vi "P3 Side.vi"(0 "Image In":T1, 1 "File Path (Grid Calibration)":path=path "C:/Users/serce/Desktop/Smart Vision System Testbench/Grid Calibration.png", 2 "Template File Path (Locate P3 Hole)":path=path "C:/Users/serce/Desktop/Smart Vision System Testbench/P3 Side/P3 Side Template.png", 7 "error in":errorcluster) -> (20 "Image Out":T1, 21 "Number of Matches (Locate P3 Hole)":i32, 22 "Fitted Circle (P3 Hole)":T2 {"Average SNR (dB)" format="%.2f"; "Average Strength" format="%.2f"; "Roundness (Real-World)" format="%.2f"; "Radius (Real-World)" format="%.2f"; "Center (Real-World)"."Y" format="%.2f"; "Center (Real-World)"."X" format="%.2f"; "Radius (Pixels)" format="%.2f"; "Center (Pixels)"."Y" format="%.2f"; "Center (Pixels)"."X" format="%.2f"}, 23 "Calibrated Results (P3 Side Top Length)":sgl[][](array[numeric]) format="%.2f", 27 "error out":errorcluster)   [LabVIEW 2020]
uses:
  <vilib>/vision/Image Controls.llb/IMAQ Image.ctl
  <vilib>/vision/Pattern Matching.llb/IMAQ Curve Parameters.ctl
  <vilib>/vision/Pattern Matching.llb/IMAQ Match Range Setting.ctl
  <vilib>/vision/Pattern Matching.llb/IMAQ Geometric Pattern 2 Advanced Match Options.ctl
  <vilib>/vision/Image Controls.llb/Vision Info Type2.ctl
  <vilib>/vision/Measure.llb/Edge Options.ctl
  <vilib>/vision/Measure.llb/Edge Polarity.ctl
  <vilib>/vision/NI_Vision_Development_Module.lvlib
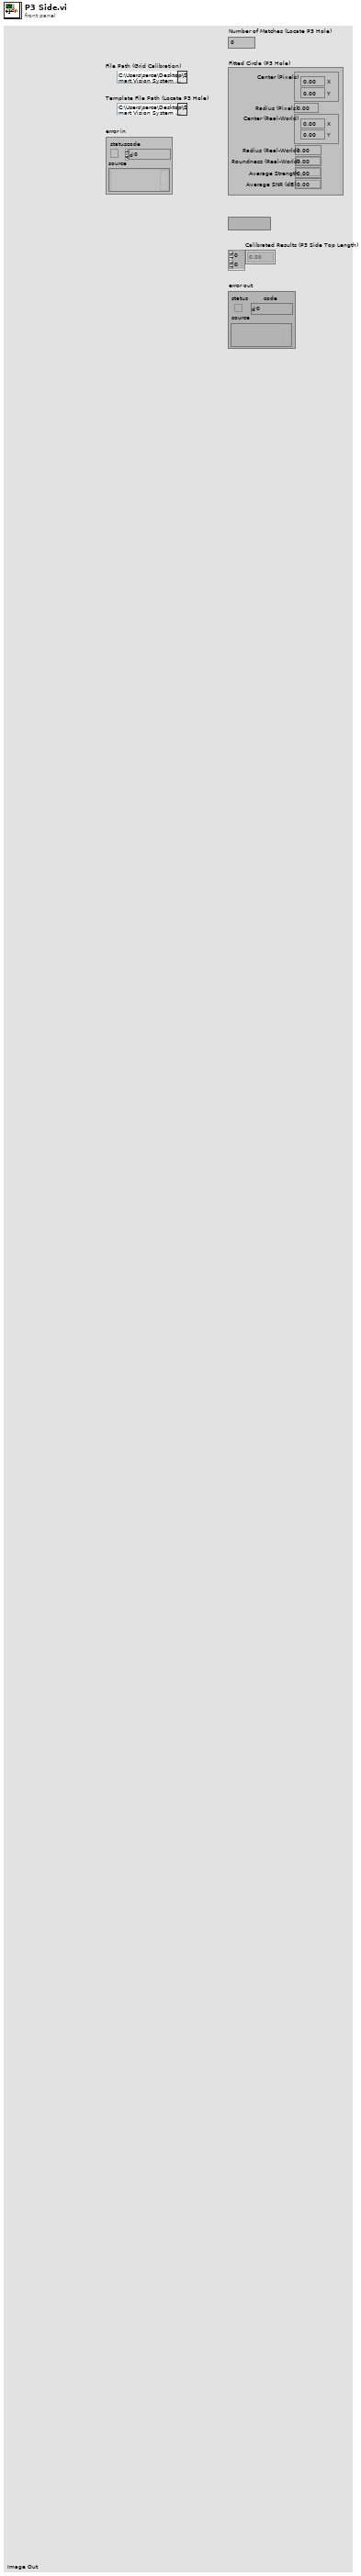
[diagram p1: front panel]
types:
  T1 = typedef "IMAQ Image.ctl" = refnum<image>
  T2 = cluster{"Center (Pixels)":cluster{"X":sgl, "Y":sgl}, "Radius (Pixels)":dbl, "Center (Real-World)":cluster{"X":sgl, "Y":sgl}, "Radius (Real-World)":dbl, "Roundness (Real-World)":dbl, "Average Strength":dbl, "Average SNR (dB)":dbl}
  T3 = cluster{"Feature":u32, "Points IDs":cluster{"GUID":string, "Index":i32}[]}[]
  T4 = cluster{"Edge Polarity":u32, "Kernel Size":u32, "Width":u32, "Minimum Edge Strength":sgl, "Interpolation Type":enum32{"Zero Order", "Bilinear", "Quadratic", "Cubic", "Bilinear Fixed"}, "Data Processing Method":enum32{"Average", "Median"}}
  T5 = enum16{"Get First Edge", "Get First + Last Edge", "Get All Edges", "Get Best Edge"}
  T6 = cluster{"Global Rectangle":i32[], "Contours":cluster{"ID":enum32{"External", "Internal"}, "Type":u32, "Coordinates":i32[]}[]}
  T7 = cluster{"Origin":cluster{"X":sgl, "Y":sgl}, "Angle (deg)":sgl, "Axis Reference":u32}
  T8 = enum16{"Reset", "Update Coordinate System", "Get Coordinate System"}
  T9 = typedef "Edge Options.ctl" = cluster{"Edge Polarity":T10, "Kernel Size":u32, "Width":u32, "Minimum Edge Strength":sgl, "Interpolation Type":enum32{"Zero Order", "Bilinear", "Quadratic", "Cubic", "Bilinear Fixed"}, "Data Processing Method":enum32{"Average", "Median"}}
  T10 = typedef "Edge Polarity.ctl" = u32
  T11 = cluster{"Search  Direction":u32, "Edge Options":T9, "Show Search Area":bool, "Show Search Lines":bool, "Show Edges Found":bool, "Show Result":bool, "Search Area Color":u32, "Search Lines Color":u32, "Edge Locations Color":u32, "Result Color":u32, "Overlay Group Name":string}
  T12 = cluster{"Process":enum16{"Get First Edge", "Get First + Last Edge", "Get All Edges", "Get Best Edge"}, "Step Size":i32, "Max Pixel Radius":i32}
  T13 = cluster{"Origin Pixel":cluster{"X":sgl, "Y":sgl}, "X Axis Pixel":cluster{"X":sgl, "Y":sgl}, "Axis Reference":u32}
  T14 = typedef "Vision Info Type2.ctl" = u32
  T15 = typedef "Simple Grid Descriptor" = cluster{"X Step":sgl, "Y Step":sgl, "Unit":T16}
  T16 = typedef "Image Unit" = enum32{"Undefined", "Angström", "Micrometer", "Millimeter", "Centimeter", "Meter", "Kilometer", "Microinch", "Inch", "Feet", "Nautical miles", "Standard miles", "Steps"}
  T17 = enum16{"Horizontal Motion", "Vertical Motion", "Horizontal and Vertical Motion", "Horizontal, Vertical and Angular Motion"}
  T18 = typedef "IMAQ Curve Parameters.ctl" = cluster{"Extraction Mode":u32, "Edge Threshold":i32, "Edge Filter Size":u32, "Min Length":i32, "Row Search Step Size":i32, "Col Search Step Size":i32, "Max Endpoint Gap":i32, "Closed":bool, "Subpixel":bool}
  T19 = typedef "IMAQ Match Range Setting.ctl" = cluster{"Match Constraints":u32, "Min":dbl, "Max":dbl}
  T20 = typedef "IMAQ Geometric Pattern 2 Advanced Match Options.ctl" = u16
  T21 = cluster{"Curve Parameters":T18, "Match Mode":cluster{"Rotation":bool, "Scale":bool, "Occlusion":bool, "Reserved 1":bool, "Reserved 2":bool, "Reserved 3":bool}, "Range Settings":T19[], "Number of Matches":i32, "Minimum Match Score":sgl, "SubPixel Accuracy":bool, "Adv. Geometric Match Options 2":cluster{"Setup Data Item":T20, "Item Value":dbl}[]}
  T22 = cluster{"Brightness":sgl, "Contrast":sgl, "Gamma":sgl}
  T23 = typedef "IMAQ GM Match Report.ctl" = cluster{"Position":cluster{"x":sgl, "y":sgl}, "Angle":sgl, "Scale":sgl, "Score":sgl, "Bounding Box":cluster{"x":sgl, "y":sgl}[], "Contrast Reversed":bool, "Occlusion %":sgl, "Template Target Curve Score":sgl, "Target Template Curve Score":sgl, "Correlation Score":sgl}
  T24 = typedef "IMAQ Coordinate System" = cluster{"Reference System":cluster{"Origin":cluster{"X":sgl, "Y":sgl}, "Angle (deg)":sgl, "Axis Reference":u32}, "Measurement System":cluster{"Origin":cluster{"X":sgl, "Y":sgl}, "Angle (deg)":sgl, "Axis Reference":u32}}
  T25 = typedef "ROI Descriptor" = cluster{"Global Rectangle":i32[], "Contours":cluster{"ID":enum32{"External", "Internal"}, "Type":u32, "Coordinates":i32[]}[]}
  T26 = typedef "Edge New.ctl" = cluster{"Location (Pixel)":cluster{"X":sgl, "Y":sgl}, "Location (Real-World)":cluster{"X":sgl, "Y":sgl}, "Distance (Pixel)":dbl, "Distance (Real-World)":dbl, "Strength":dbl, "Noise":dbl, "Rising?":bool}
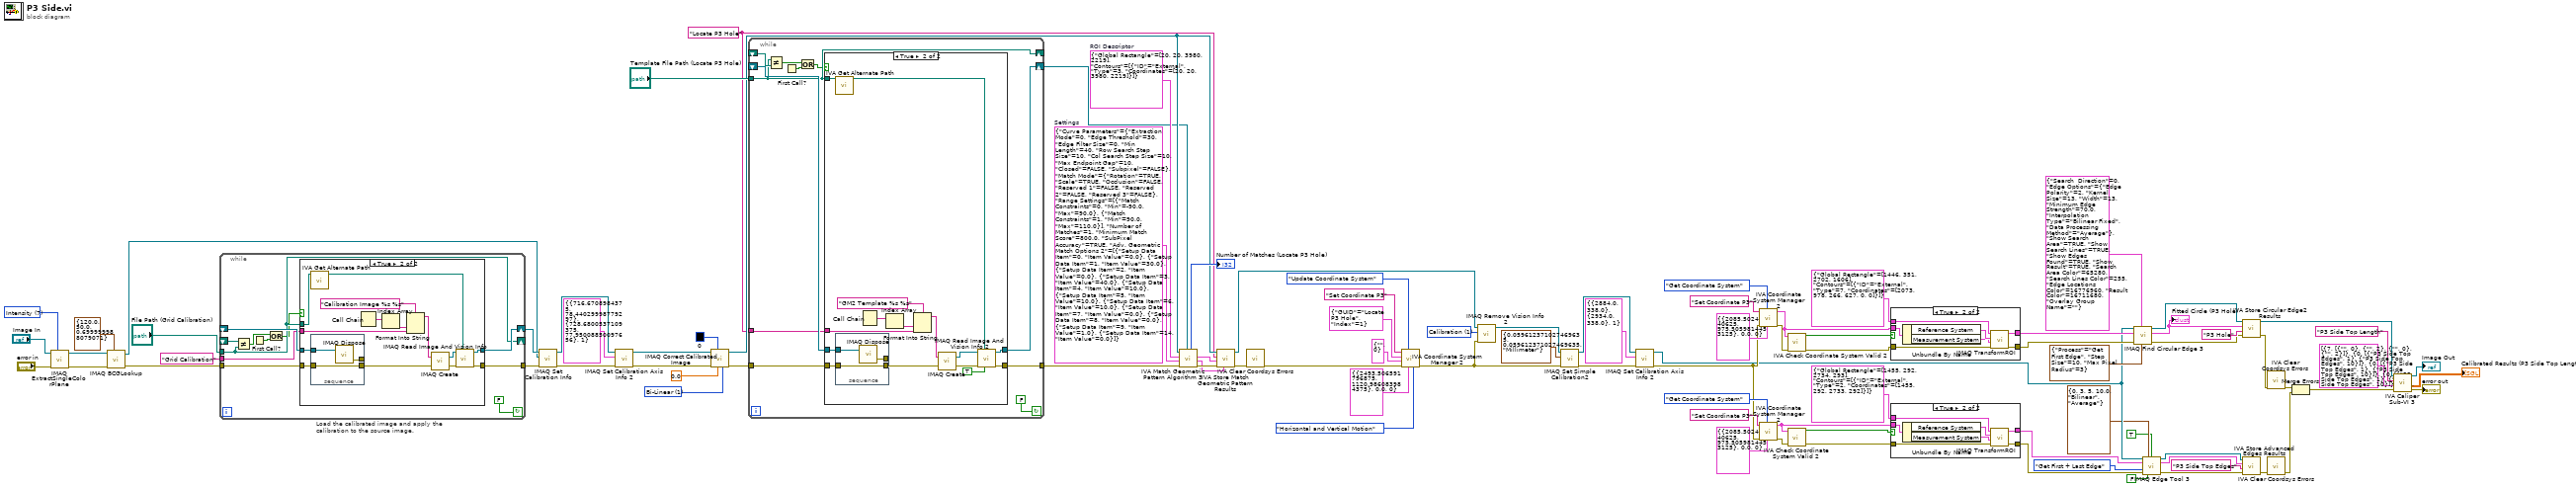
[diagram p0: block diagram]
diagram:
  w54 = T14 1 items=["Any", "Calibration", "Overlay", "Grayscale Template", "Color Template", "Geometric Template", "Custom Data", "Golden Template", "Geometric Template 2", "Contour Data", "Camera Model"] ("Vision Info")
  w67 = T21 {"Curve Parameters"={"Extraction Mode"=0, "Edge Threshold"=30, "Edge Filter Size"=0, "Min Length"=40, "Row Search Step Size"=10, "Col Search Step Size"=10, "Max Endpoint Gap"=10, "Closed"=FALSE, "Subpixel"=FALSE}, "Match Mode"={"Rotation"=TRUE, "Scale"=TRUE, "Occlusion"=FALSE, "Reserved 1"=FALSE, "Reserved 2"=FALSE, "Reserved 3"=FALSE}, "Range Settings"=[{"Match Constraints"=0, "Min"=-90.0, "Max"=90.0}, {"Match Constraints"=1, "Min"=90.0, "Max"=110.0}], "Number of Matches"=1, "Minimum Match Score"=800.0, "SubPixel Accuracy"=TRUE, "Adv. Geometric Match Options 2"=[{"Setup Data Item"=0, "Item Value"=0.0}, {"Setup Data Item"=1, "Item Value"=30.0}, {"Setup Data Item"=2, "Item Value"=0.0}, {"Setup Data Item"=3, "Item Value"=40.0}, {"Setup Data Item"=4, "Item Value"=10.0}, {"Setup Data Item"=5, "Item Value"=10.0}, {"Setup Data Item"=6, "Item Value"=10.0}, {"Setup Data Item"=7, "Item Value"=0.0}, {"Setup Data Item"=8, "Item Value"=0.0}, {"Setup Data Item"=9, "Item Value"=1.0}, {"Setup Data Item"=14, "Item Value"=0.0}]}  # Settings
  w66 = "Locate P3 Hole" ("Step Name")
  w74 = T6 {"Global Rectangle"=[20, 20, 3980, 2219], "Contours"=[{"ID"=enum."External", "Type"=3, "Coordinates"=[20, 20, 3980, 2219]}]}  # ROI Descriptor
  w80 = u32 1 items=["Zero Order", "Bi-Linear", "Quadratic", "Cubic Spline"] ("Interpolation Type")
  w95 = 7 items=["Red", "Green", "Blue", "Hue", "Saturation", "Luminance", "Value", "Intensity"] ("Color Plane")
  n1 = call "IMAQ ExtractSingleColorPlane"("Color Plane"=w95, "error in (no error)"="error in", "Image Src"="Image In") -> ("error out"=w91:errorcluster, "Image Dst Out"=w92:T1)  [unwired: 1 in, 6 out]
  n2 = call "IMAQ BCGLookup"("Image Src"=w92, "BCG Values"=T22 {"Brightness"=120.0, "Contrast"=50.0, "Gamma"=0.7}, "error in (no error)"=w91) -> ("Image Dst Out"=w85:T1, "error out"=w89:errorcluster)  [unwired: 2 in, 2 out]
  n3 = while "Load the calibrated image and apply the calibration to the source image." {
    shift-right: [w106] -> w87
    shift-left: _ -> [w105]
    tunnel: [w103] -> w86
    tunnel: w89 -> [w102]
    tunnel: "File Path (Grid Calibration)" -> [w99]
    tunnel: "Grid Calibration" ("Step Name") -> [w101]
    shift-right: [w99] -> _
    shift-left: _ -> [w100]
    stop <- FALSE continue-if-true
    n4 = Not Equal?(x=w100, y=w99) -> (x != y?=w97:bool)
    n5 = First Call?() -> (First Call?: T/F=w98:bool)
    n6 = Or(x=w97, y=w98) -> (x .or. y?=w96:bool)
    n7 = case shown="True" w96 {
      tunnel: [w108 w120] -> w106
      tunnel: w105 -> [w108 w112]
      tunnel: [w107 w117] -> w103
      tunnel: w102 -> [w107 w113]
      tunnel: w99 -> [_ w110]
      tunnel: w101 -> [_ w114]
      frame False {
      }
      frame True {
        n8 = call <vilib>:"IVA Get Alternate Path.vi"("Path In"=w110) -> ("Path Out"=w109:path)  [unwired: 10 out]
        n9 = stacked-sequence {
          tunnel: w113 -> [w124]
          tunnel: w112 -> [w125]
          tunnel: [w124] -> w111
          tunnel: [w123] -> _
          frame #0 {
            n10 = call "IMAQ Dispose"("Image"=w125) -> ("error out"=w123:errorcluster)  [unwired: 2 in, 3 out]
          }
        }
        n11 = Call Chain() -> (call chain=w116:string[])
        n12 = Index Array(array=w116) -> (element=w115:string)  [unwired: 1 in]
        n13 = Format Into String(format string="Calibration Image %s %s" ("Image Name"), w115, w114) -> (resulting string=w122:string)  [unwired: 2 in, 1 out]
        n14 = call "IMAQ Create"("Image Name"=w122, "error in (no error)"=w111) -> ("New Image"=w119:T1, "error out"=w118:errorcluster)  [unwired: 2 in, 1 out]
        n15 = call "IMAQ Read Image And Vision Info"("File Path"=w109, "error in (no error)"=w118, "Image"=w119) -> ("error out"=w117:errorcluster, "Image Out"=w120:T1)  [unwired: 1 in, 6 out]
      }
    }
  }
  n16 = call "IMAQ Set Calibration Info"("error in (no error)"=w86, "Image Dst"=w85, "Image Src"=w87) -> ("error out"=w82:errorcluster, "Calibrated Image"=w83:T1)  [unwired: 1 in, 6 out]
  n17 = call-poly "IMAQ Set Calibration Axis Info 2"("error in (no error)"=w82, "Calibration Axis Info"=T13 {"Origin Pixel"={"X"=716.6709, "Y"=78.4403}, "X Axis Pixel"={"X"=728.68005, "Y"=77.95009}, "Axis Reference"=1}, "Calibration Template Image In"=w83) -> ("error out"=w78:errorcluster, "Calibration Template Image Out"=w79:T1)  [unwired: 7 out]
  n18 = call "IMAQ Correct Calibrated Image"("Interpolation Type"=w80, "Replace Value"=sgl 0.0, "Color Replace Value"=u32 0, "error in (no error)"=w78, "Image Src"=w79) -> ("error out"=w69:errorcluster, "Corrected Image"=w68:T1)  [unwired: 2 in, 3 out]
  n19 = while {
    shift-right: [w136] -> w64
    shift-left: _ -> [w135]
    tunnel: [w133] -> w65
    tunnel: w69 -> [w132]
    tunnel: "Template File Path (Locate P3 Hole)" -> [w129]
    tunnel: w66 -> [w131]
    shift-right: [w129] -> _
    shift-left: _ -> [w130]
    stop <- FALSE continue-if-true
    n20 = Not Equal?(x=w129, y=w130) -> (x != y?=w127:bool)
    n21 = First Call?() -> (First Call?: T/F=w128:bool)
    n22 = Or(x=w127, y=w128) -> (x .or. y?=w126:bool)
    n23 = case shown="True" w126 {
      tunnel: [w138 w140] -> w136
      tunnel: w135 -> [w138 w147]
      tunnel: [w137 w142] -> w133
      tunnel: w132 -> [w137 w148]
      tunnel: w131 -> [_ w149]
      tunnel: w129 -> [_ w146]
      frame False {
      }
      frame True {
        n24 = call <vilib>:"IVA Get Alternate Path.vi"("Path In"=w146) -> ("Path Out"=w141:path)  [unwired: 10 out]
        n25 = stacked-sequence {
          tunnel: w148 -> [w156]
          tunnel: w147 -> [w155]
          tunnel: [w156] -> w145
          tunnel: [w154] -> _
          frame #0 {
            n26 = call "IMAQ Dispose"("Image"=w155) -> ("error out"=w154:errorcluster)  [unwired: 2 in, 3 out]
          }
        }
        n27 = Call Chain() -> (call chain=w151:string[])
        n28 = Index Array(array=w151) -> (element=w150:string)  [unwired: 1 in]
        n29 = Format Into String(format string="GM2 Template %s %s" ("Image Name"), w150, w149) -> (resulting string=w153:string)  [unwired: 2 in, 1 out]
        n30 = call "IMAQ Create"("Image Name"=w153, "error in (no error)"=w145) -> ("New Image"=w139:T1, "error out"=w143:errorcluster)  [unwired: 2 in, 1 out]
        n31 = call "IMAQ Read Image And Vision Info 2"("Use File Path Image Type"=TRUE, "File Path"=w141, "error in (no error)"=w143, "Image"=w139) -> ("error out"=w142:errorcluster, "Image Out"=w140:T1)  [unwired: 5 in, 1 out]
      }
    }
  }
  n32 = call <vilib>:"IVA Match Geometric Pattern Algorithm 3.vi"("Template"=w64, "error in (no error)"=w65, "Settings"=w67, "ROI Descriptor"=w74, "Image"=w68) -> ("error out"=w73:errorcluster, "Calibrated Matches"=w71:T23[], "Matches"=w72:T23[], "Number of Matches"=→"Number of Matches (Locate P3 Hole)":i32)  [unwired: 3 out]
  n33 = call <vilib>:"IVA Store Match Geometric Pattern Results.vi"("Calibrated Matches"=w71, "error in (no error)"=w73, "Matches"=w72, "Step Name"=w66, "Image in"=w68) -> ("error out"=w63:errorcluster, "Image dup"=w53:T1)  [unwired: 5 out]
  n34 = call <vilib>:"IVA Clear Coordsys Errors.vi"("error in (no error)"=w63) -> ("error out"=w56:errorcluster)  [unwired: 10 in]
  n35 = call <vilib>:"IVA Coordinate System Manager 2.vi"("Mode"=T17."Horizontal and Vertical Motion", "Reference System"=T7 {"Origin"={"X"=2493.5066, "Y"=1120.9861}, "Angle (deg)"=0.0, "Axis Reference"=0}, "Function"=T8."Update Coordinate System", "error in (no error)"=w56, "Angle ID"=cluster{"GUID":string, "Index":i32} {"GUID"="", "Index"=0}, "Origin ID"=cluster{"GUID":string, "Index":i32} {"GUID"="Locate P3 Hole", "Index"=1}, "Coordinate System Name"="Set Coordinate P3") -> ("error out"=w51:errorcluster)  [unwired: 4 out]
  n36 = call "IMAQ Remove Vision Info 2"("error in (no error)"=w51, "Vision Info"=w54, "Image"=w53) -> ("Image Out"=w52:T1)  [unwired: 8 out]
  n37 = call "IMAQ Set Simple Calibration2"("error in (no error)"=w51, "Pixel Distances"=T15 {"X Step"=0.05961237, "Y Step"=0.05961237, "Unit"=enum."Millimeter"} ("Grid Descriptor"), "Image"=w52) -> ("error out"=w49:errorcluster, "Calibration Template Image"=w50:T1)  [unwired: 2 in, 5 out]
  n38 = call-poly "IMAQ Set Calibration Axis Info 2"("error in (no error)"=w49, "Calibration Axis Info"=T13 {"Origin Pixel"={"X"=2884.0, "Y"=338.0}, "X Axis Pixel"={"X"=2934.0, "Y"=338.0}, "Axis Reference"=1}, "Calibration Template Image In"=w50) -> ("error out"=w28:errorcluster, "Calibration Template Image Out"=w21:T1)  [unwired: 7 out]
  n39 = call <vilib>:"IVA Coordinate System Manager 2.vi"("Reference System"=T7 {"Origin"={"X"=2085.5024, "Y"=975.506}, "Angle (deg)"=0.0, "Axis Reference"=0}, "Function"=T8."Get Coordinate System", "error in (no error)"=w28, "Coordinate System Name"="Set Coordinate P3") -> ("error out"=w41:errorcluster, "Coordinate System Out"=w43:T24)  [unwired: 3 in, 3 out]
  n40 = call <vilib>:"IVA Coordinate System Manager 2.vi"("Reference System"=T7 {"Origin"={"X"=2085.5024, "Y"=975.506}, "Angle (deg)"=0.0, "Axis Reference"=0}, "Function"=T8."Get Coordinate System", "error in (no error)"=w28, "Coordinate System Name"="Set Coordinate P3") -> ("error out"=w23:errorcluster, "Coordinate System Out"=w25:T24)  [unwired: 3 in, 3 out]
  n41 = call <vilib>:"IVA Check Coordinate System Valid 2.vi"("error in (no error)"=w41, "Coordinate System"=w43) -> ("error out"=w40:errorcluster, "Valid?"=w42:bool)  [unwired: 8 out]
  n42 = call <vilib>:"IVA Check Coordinate System Valid 2.vi"("error in (no error)"=w23, "Coordinate System"=w25) -> ("error out"=w22:errorcluster, "Valid?"=w24:bool)  [unwired: 8 out]
  n43 = case shown="True" w42 {
    tunnel: T6 {"Global Rectangle"=[1446, 351, 2702, 1606], "Contours"=[{"ID"=enum."External", "Type"=7, "Coordinates"=[2073, 978, 266, 627, 0, 0]}]} ("ROI Descriptor") -> [w158 w165]
    tunnel: [w158 w162] -> w38
    tunnel: [w157 w161] -> w37
    tunnel: w43 -> [_ w160]
    tunnel: w40 -> [w157 w159]
    frame False {
    }
    frame True {
      n44 = Unbundle By Name(w160) -> ("Reference System"=w164:T7, "Measurement System"=w163:T7)
      n45 = call "IMAQ TransformROI"("error in (no error)"=w159, "New Reference"=w163, "Base Reference"=w164, "ROI Descriptor"=w165) -> ("error out"=w161:errorcluster, "ROI Descriptor out"=w162:T25)  [unwired: 6 out]
    }
  }
  n46 = case shown="True" w24 {
    tunnel: T6 {"Global Rectangle"=[1455, 292, 2734, 293], "Contours"=[{"ID"=enum."External", "Type"=2, "Coordinates"=[1455, 292, 2733, 292]}]} ("ROI Descriptor") -> [w167 w174]
    tunnel: [w167 w171] -> w14
    tunnel: [w166 w170] -> w13
    tunnel: w25 -> [_ w169]
    tunnel: w22 -> [w166 w168]
    frame False {
    }
    frame True {
      n47 = Unbundle By Name(w169) -> ("Reference System"=w173:T7, "Measurement System"=w172:T7)
      n48 = call "IMAQ TransformROI"("error in (no error)"=w168, "New Reference"=w172, "Base Reference"=w173, "ROI Descriptor"=w174) -> ("error out"=w170:errorcluster, "ROI Descriptor out"=w171:T25)  [unwired: 6 out]
    }
  }
  n49 = call "IMAQ Find Circular Edge 3"("Circle Fit Options"=T12 {"Process"=enum."Get First Edge", "Step Size"=10, "Max Pixel Radius"=3}, "Options"=T11 {"Search  Direction"=0, "Edge Options"={"Edge Polarity"=2, "Kernel Size"=13, "Width"=13, "Minimum Edge Strength"=70.0, "Interpolation Type"=enum."Bilinear Fixed", "Data Processing Method"=enum."Average"}, "Show Search Area"=TRUE, "Show Search Lines"=TRUE, "Show Edges Found"=TRUE, "Show Result"=TRUE, "Search Area Color"=65280, "Search Lines Color"=255, "Edge Locations Color"=16776960, "Result Color"=16711680, "Overlay Group Name"=""}, "error in (no error)"=w37, "ROI Descriptor"=w38, "Image"=w21) -> ("error out"=w33:errorcluster, "Fitted Circle"=w35:T2, "Image Out"=w32:T1)  [unwired: 2 in, 2 out]
  "Fitted Circle (P3 Hole)" <- w35
  n50 = call "IMAQ Edge Tool 3"("Image"=w21, "Edge Options"=T4 {"Edge Polarity"=0, "Kernel Size"=3, "Width"=5, "Minimum Edge Strength"=10.0, "Interpolation Type"=enum."Bilinear", "Data Processing Method"=enum."Average"}, "Optimized Mode"=TRUE, "ROI Descriptor"=w14, "Process"=T5."Get First + Last Edge", "error in (no error)"=w13, "Reverse Direction"=FALSE) -> ("Image (duplicate)"=w17:T1, "Edge Information"=w16:T26[], "error out"=w18:errorcluster)  [unwired: 6 out]
  n51 = call <vilib>:"IVA Store Circular Edge2 Results.vi"("error in (no error)"=w33, "Step Name"="P3 Hole", "Fitted Circle"=w35, "Image in"=w32) -> ("error out"=w31:errorcluster, "Image dup"=w7:T1)  [unwired: 2 in, 4 out]
  n52 = call <vilib>:"IVA Store Advanced Edges Results.vi"("error in (no error)"=w18, "Step Name"="P3 Side Top Edges", "Edge Information"=w16, "Image in"=w17) -> ("error out"=w10:errorcluster)  [unwired: 7 out]
  n53 = call <vilib>:"IVA Clear Coordsys Errors.vi"("error in (no error)"=w31) -> ("error out"=w9:errorcluster)  [unwired: 10 in]
  n54 = call <vilib>:"IVA Clear Coordsys Errors.vi"("error in (no error)"=w10) -> ("error out"=w8:errorcluster)  [unwired: 10 in]
  n55 = Merge Errors(w9, w8) -> (w6:errorcluster)
  n56 = call <vilib>:"IVA Caliper Sub-VI 3.vi"("error in"=w6, "Parameters"=T3 [{"Feature"=7, "Points IDs"=[{"GUID"="", "Index"=0}, {"GUID"="", "Index"=2}, {"GUID"="", "Index"=0}, {"GUID"="", "Index"=2}]}, {"Feature"=0, "Points IDs"=[{"GUID"="P3 Side Top Edges", "Index"=1}, {"GUID"="P3 Side Top Edges", "Index"=10}]}, {"Feature"=0, "Points IDs"=[{"GUID"="P3 Side Top Edges", "Index"=1}, {"GUID"="P3 Side Top Edges", "Index"=10}]}, {"Feature"=0, "Points IDs"=[{"GUID"="P3 Side Top Edges", "Index"=1}, {"GUID"="P3 Side Top Edges", "Index"=10}]}, {"Feature"=0, "Points IDs"=[{"GUID"="P3 Side Top Edges", "Index"=1}, {"GUID"="P3 Side Top Edges", "Index"=10}]}], "Step Name"="P3 Side Top Length", "Image In"=w7) -> ("error out"=→"error out":errorcluster, "Results (Calibrated)"=→"Calibrated Results (P3 Side Top Length)":sgl[][], "Image Out"=→"Image Out":T1)  [unwired: 1 in, 4 out]
